vi "UE9 Single EI-1050 Example.vi"() -> ()   [LabVIEW 2021]
panel:
  in  "stop":bool
  out "ms per iteration":u32
  out "RH A [%]":dbl format="%.6f"
  out "Temp A [degC]":dbl format="%.6f"
  out "Error Message":string
  out "error out":errorcluster
  # "Reads temperature and humidity from an EI-1050 probe:\n\nEI-1050 Connections:\nRed (Power)         FIO2\nBlack (Ground)     GND\nGreen (Data)        FIO0\nWhite (Clock)       FIO1\nBrown (Enable)    FIO2"
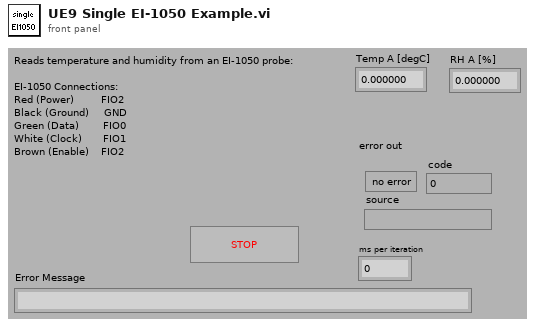
[diagram p1: front panel]
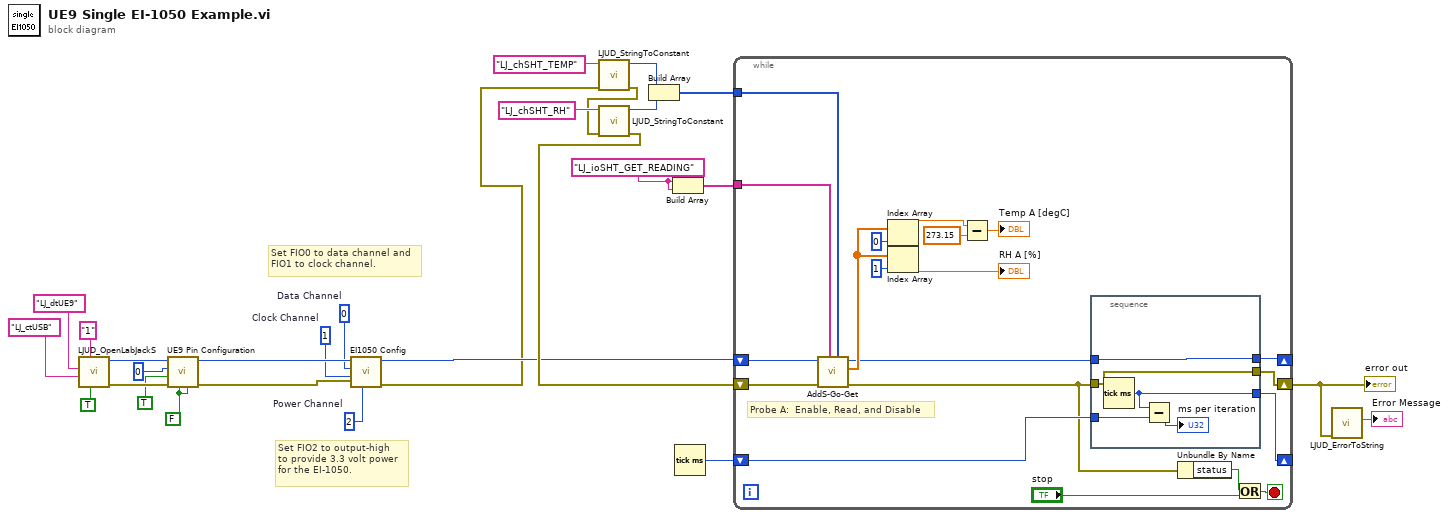
[diagram p0: block diagram]
diagram:
  w3 = 2  # Power Channel
  w4 = 1  # Clock Channel
  w5 = 0  # Data Channel
  w9 = FALSE ("Enable DAC1")
  w20 = "LJ_ioSHT_GET_READING" ("IOType")
  # "Set FIO2 to output-high\nto provide 3.3 volt power\nfor the EI-1050."
  # "Set FIO0 to data channel and\nFIO1 to clock channel."
  n1 = call "LJUD_OpenLabJackS.vi"("FirstFound"=TRUE, "Address"="1", "ConnectionType"="LJ_ctUSB", "DeviceType"="LJ_dtUE9") -> ("error out"=w22:errorcluster, "Handle"=w23:i32)  [unwired: 5 in, 1 out]
  n2 = call "UE9 Pin Configuration.vi"("Enable Counter1"=w9, "Enable Counter0"=w9, "error in"=w22, "Enable DACs"=TRUE ("Enable DAC1"), "Number of Timers Enabled"=u8 0, "Handle In"=w23) -> ("error out"=w6:errorcluster, "Handle Out"=w7:i32)  [unwired: 4 in]
  n3 = call "EI1050 Config.vi"("Power Channel"=w3, "error in"=w6, "Clock Channel"=w4, "Data Channel"=w5, "Handle In"=w7) -> ("error out"=w1:errorcluster, "Handle Out"=w2:i32)  [unwired: 5 in]
  n4 = call "LJUD_StringToConstant.vi"("error in"=w1, "String"="LJ_chSHT_TEMP") -> ("error out"=w11:errorcluster, "Constant Number"=w19:i32)  [unwired: 8 in]
  n5 = call "LJUD_StringToConstant.vi"("error in"=w11, "String"="LJ_chSHT_RH") -> ("error out"=w10:errorcluster, "Constant Number"=w18:i32)  [unwired: 8 in]
  n6 = Build Array(w19, w18) -> (w14:i32[])
  n7 = Build Array(w20, w20) -> (w15:string[])
  n8 = Tick Count (ms)() -> (millisecond timer value=w13:u32)
  n9 = while {
    shift-left: w13 -> [w38]
    shift-right: [w41] -> _
    shift-left: w2 -> [w30]
    shift-right: [w39] -> _
    shift-left: w10 -> [w29]
    shift-right: [w40] -> w12
    tunnel: w14 -> [w34]
    tunnel: w15 -> [w33]
    stop <- w37 stop-if-true
    # "Probe A:  Enable, Read, and Disable"
    n10 = call "AddS-Go-Get.vi"("Channels"=w34, "IOTypes"=w33, "error in"=w29, "Handle In"=w30) -> ("error out"=w31:errorcluster, "Values Read"=w46:dbl[], "Handle Out"=w32:i32)  [unwired: 5 in]
    n11 = Index Array(array=w46, index=0 ("Index")) -> (element=w43:dbl)
    n12 = Index Array(array=w46, index=1 ("Index")) -> (element=→"RH A [%]":dbl)
    n13 = Subtract(x=w43, y=273.15) -> (x-y=→"Temp A [degC]":dbl)
    n14 = stacked-sequence {
      tunnel: [w53] -> w41
      tunnel: w31 -> [w52]
      tunnel: [w52] -> w40
      tunnel: [w51] -> w39
      tunnel: w32 -> [w51]
      tunnel: w38 -> [w50]
      frame #0 {
        n15 = Tick Count (ms)() -> (millisecond timer value=w53:u32)
        n16 = Subtract(x=w53, y=w50) -> (x-y=→"ms per iteration":u32)
      }
    }
    n17 = Unbundle By Name(w31) -> ("status"=w36:bool)
    n18 = Or(x=w36, y="stop") -> (x .or. y?=w37:bool)
  }
  "error out" <- w12
  n19 = call "LJUD_ErrorToString.vi"("error in"=w12) -> ("String"=→"Error Message":string)  [unwired: 10 in]
